vi "SimpleSerialTest.vi"() -> ()   [LabVIEW 2013]
uses:
  Data/TypeDefs/Notifiers.ctl
  Data/TypeDefs/UTM Location.ctl
  Data/TypeDefs/Sail Set Suggestions.ctl
  Data/TypeDefs/Rudder Set Suggestions.ctl
  Data/TypeDefs/OverrideInformation.ctl
  Data/TypeDefs/OverrideMode.ctl
  Data/TypeDefs/MotorSetup.ctl
  Data/TypeDefs/DynamixelSetupInfo.ctl
  Data/TypeDefs/AirmarStatus.ctl
  Data/TypeDefs/HardwareOnline.ctl
  Data/TypeDefs/DynamixelCycleTracker.ctl
  Data/TypeDefs/RC Input Values.ctl
  Classes/Waypoint/Waypoint.lvclass
  Data/TypeDefs/GPS-Compass Queue Cluster.ctl
  <vilib>/Instr/_visa.llb/VISA Configure Serial Port (Instr).vi
  Data/TypeDefs/WindData Queue Cluster.ctl
panel:
  out "Sentence":string
  in  "stop":bool
  out "While counter":i32
  in  "NotifierReff":T1
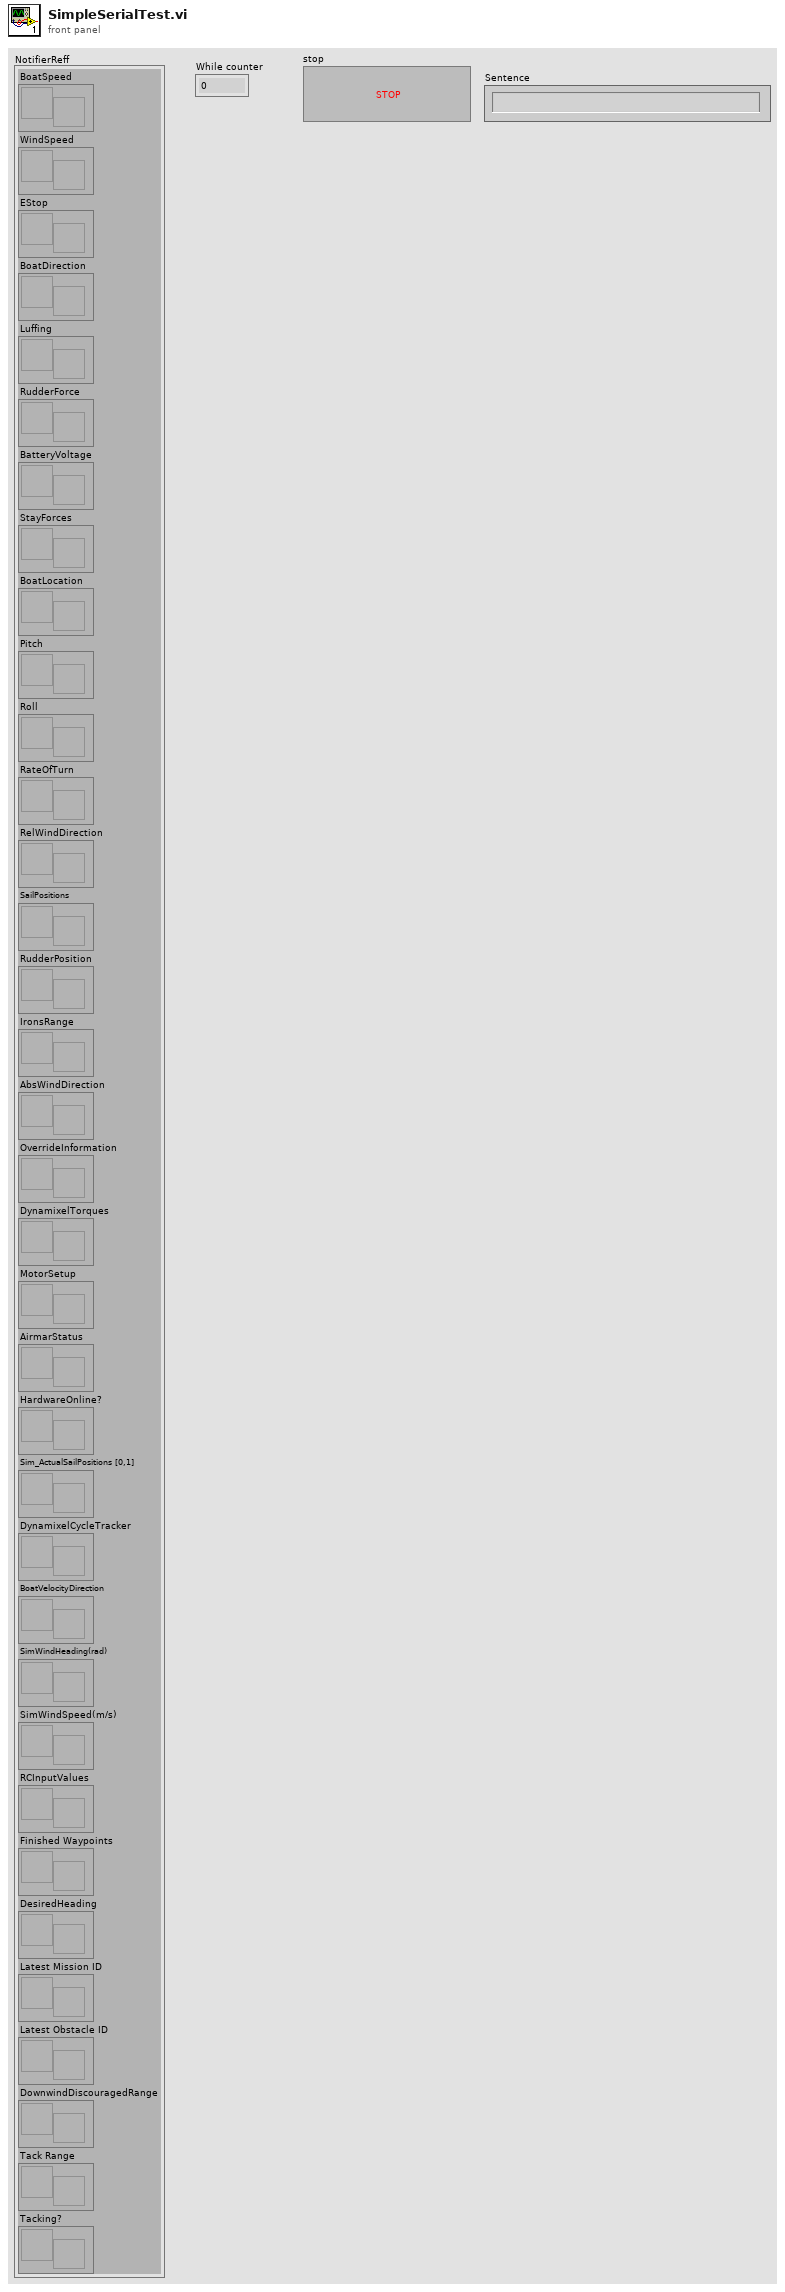
[diagram p1: front panel]
types:
  T1 = typedef "Notifiers.ctl" = cluster{"BoatSpeed":refnum<notifier>, "WindSpeed":refnum<notifier>, "EStop":refnum<notifier>, "BoatDirection":refnum<notifier>, "Luffing":refnum<notifier>, "RudderForce":refnum<notifier>, "BatteryVoltage":refnum<notifier>, "StayForces":refnum<notifier>, "BoatLocation":refnum<notifier>, "Pitch":refnum<notifier>, "Roll":refnum<notifier>, "RateOfTurn":refnum<notifier>, "RelWindDirection":refnum<notifier>, "SailPositions":refnum<notifier>, "RudderPosition":refnum<notifier>, "IronsRange":refnum<notifier>, "AbsWindDirection":refnum<notifier>, "OverrideInformation":refnum<notifier>, "DynamixelTorques":refnum<notifier>, "MotorSetup":refnum<notifier>, "AirmarStatus":refnum<notifier>, "HardwareOnline?":refnum<notifier>, "Sim_ActualSailPositions [0,1]":refnum<notifier>, "DynamixelCycleTracker":refnum<notifier>, "BoatVelocityDirection":refnum<notifier>, "SimWindHeading(rad)":refnum<notifier>, "SimWindSpeed(m/s)":refnum<notifier>, "RCInputValues":refnum<notifier>, "Finished Waypoints":refnum<notifier>, "DesiredHeading":refnum<notifier>, "Latest Mission ID":refnum<notifier>, "Latest Obstacle ID":refnum<notifier>, "DownwindDiscouragedRange":refnum<notifier>, "Tack Range":refnum<notifier>, "Tacking?":refnum<notifier>}
  T2 = typedef "WindData Queue Cluster.ctl" = cluster{"RelWindDirection Queue":refnum<queue>, "WindSpeed Queue":refnum<queue>, "AbsWindDirection Queue":refnum<queue>}
  T3 = typedef "GPS-Compass Queue Cluster.ctl" = cluster{"BoatLocation Queue":refnum<queue>, "BoatDirection Queue":refnum<queue>, "BoatSpeed Queue":refnum<queue>, "RateOfTurn Queue":refnum<queue>, "Pitch Queue":refnum<queue>, "Roll Queue":refnum<queue>, "BoatVelocityDirection Queue ":refnum<queue>}
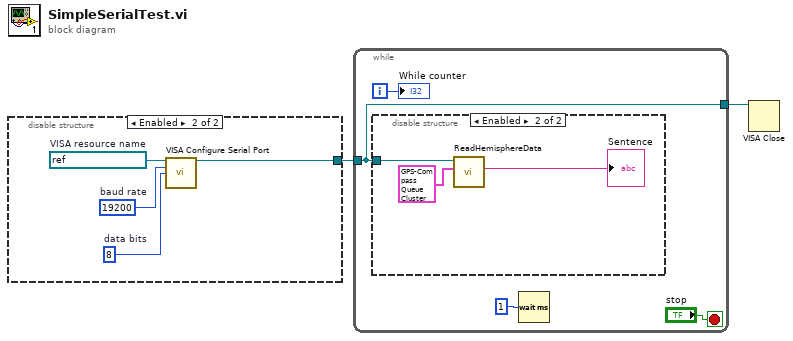
[diagram p0: block diagram]
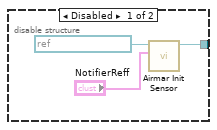
[diagram p2: hidden frame]
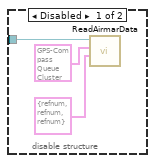
[diagram p3: hidden frame]
diagram:
  n1 = disable-structure shown="Enabled" {
    disable-tunnel: [w3 w6] -> w2
    frame Disabled {
      n2 = call "Airmar Init Sensor.vi"("NotifierReff"="NotifierReff", "VISA Refnum in"=refnum<visa-resource-name> "ASRL2::INSTR") -> ("VISA Refnum out"=w3:refnum<visa-resource-name>)  [unwired: 7 in, 2 out]
    }
    frame Enabled {
      w9 = u16 8  # data bits
      w7 = u32 19200  # baud rate
      w8 = refnum<visa-resource-name> "ASRL1::INSTR"  # VISA resource name
      n3 = call-poly "VISA Configure Serial Port"("VISA resource name"=w8, "baud rate (9600)"=w7, "data bits (8)"=w9) -> ("VISA resource name out"=w6:refnum<visa-resource-name>)  [unwired: 11 in, 1 out]
    }
  }
  n4 = while {
    tunnel: w2 -> [w10]
    tunnel: [w10] -> w1
    i -> [w13]
    stop <- "stop" stop-if-true
    n5 = disable-structure shown="Enabled" {
      disable-tunnel: w10 -> [w16 w19]
      frame Disabled {
        n6 = call "ReadAirmarData.vi"("Airmar Wind Queue Cluster"=T2 {"RelWindDirection Queue"=refnum, "WindSpeed Queue"=refnum, "AbsWindDirection Queue"=refnum}, "AirmarGPS-Compass Queue Cluster"=T3 {"BoatLocation Queue"=refnum, "BoatDirection Queue"=refnum, "BoatSpeed Queue"=refnum, "RateOfTurn Queue"=refnum, "Pitch Queue"=refnum, "Roll Queue"=refnum, "BoatVelocityDirection Queue "=refnum}, "VISA UART port"=w16) -> ()  [unwired: 7 in, 2 out]
      }
      frame Enabled {
        n7 = call "ReadHemisphereData.vi"("Hemisphere Queue Cluster"=T3 {"BoatLocation Queue"=refnum, "BoatDirection Queue"=refnum, "BoatSpeed Queue"=refnum, "RateOfTurn Queue"=refnum, "Pitch Queue"=refnum, "Roll Queue"=refnum, "BoatVelocityDirection Queue "=refnum}, "VISA UART port"=w19) -> ("Sentence"=→"Sentence":string)  [unwired: 7 in, 2 out]
      }
    }
    n8 = Wait (ms)(milliseconds to wait=u32 1) -> ()  [unwired: 1 out]
    "While counter" <- w13
  }
  n9 = VISA Close(VISA resource name=w1) -> ()  [unwired: 1 in, 1 out]
